vi "Get Pulse State.vi"(8 "error in (no error)":errorcluster, 11 "DAQmx Lockin Digitizer Driver in":refnum<class "DAQmx Lockin Digitizer Driver.lvclass">) -> (0 "error out":errorcluster, 1 "Result ready":bool, 2 "Armed":bool, 3 "DAQmx Lockin Digitizer Driver out":refnum<class "DAQmx Lockin Digitizer Driver.lvclass">)   [LabVIEW 2021, in "DAQmx Lockin Digitizer Driver.lvclass"]
uses:
  DAQmx Lockin Digitizer Driver.lvclass
  DAQmx Lockin Digitizer Driver.lvclass/DAQmx Lockin Digitizer Driver.ctl
  DAQmx Lockin Driver/DAQmx Lockin Driver.lvclass
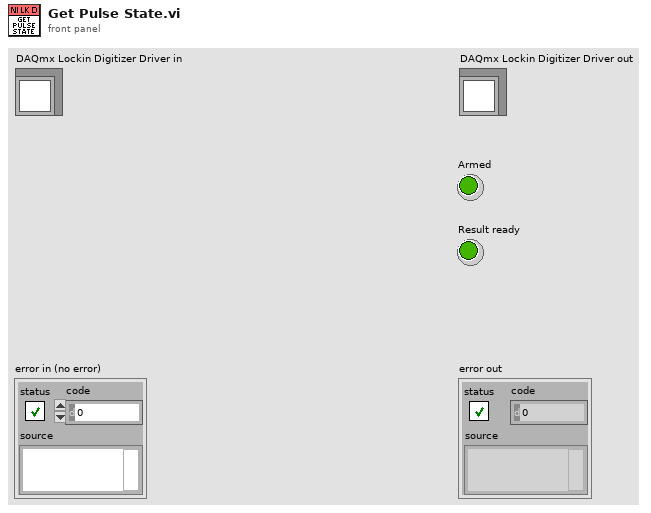
[diagram p1: front panel]
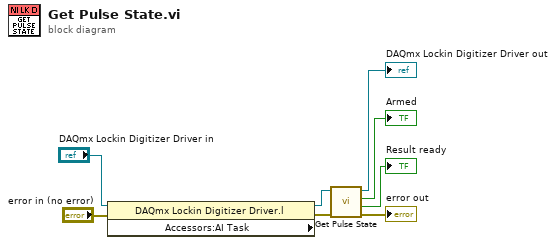
[diagram p0: block diagram]
diagram:
  n1 = property class="DAQmx Lockin Digitizer Driver.l" props=["Accessors:AI Task"](reference="DAQmx Lockin Digitizer Driver in", error in="error in (no error)") -> (reference out=w1:refnum<class "DAQmx Lockin Digitizer Driver.lvclass">, error out=w3:errorcluster)  [unwired: 1 out]
  n2 = call-parent "Get Pulse State.vi"("error in (no error)"=w3, "DAQmx Digitizer in"=w1) -> ("error out"=→"error out":errorcluster, "Result ready"=→"Result ready":bool, "Armed"=→"Armed":bool, "DAQmx Digitizer out"=→"DAQmx Lockin Digitizer Driver out":refnum<class "DAQmx Lockin Digitizer Driver.lvclass">)  [unwired: 6 in]
